vi "getLecServerCount.vi"(8 "error in (no error)":errorcluster, 11 "SM1000-control in":T1) -> (0 "error out":errorcluster, 2 "piServerCount":i32, 3 "SM1000-control out":T1)   [LabVIEW 2013, in "EC1000-control.lvlib" / "SM1000-control.lvclass"]
doc: "Get embedded controller device data.\n\nOnce a connection to the broadcast mechanism has been established, broadcast messages are then received and a table of available modules is built by the API. This method returns the number of distinct EC1000 modules that have transmitted valid broadcast packets since the 'clientAttachBroadcast' method was called.\nBecause of the asynchronous and periodic nature of the broadcast transmissions, it may take some time before all EC1000 controllers are recognized and reported via this method. Several successive calls may yield different results until enough time has passed to account for the longest broadcast interval. The broadcast interval is configured using the 'Session.requestFixedData' and 'Session.setFixedData' methods with the 'AdminConfig' data as an argument."
uses:
  SM1000-control.lvclass
  Object-reference.ctl
  SM1000-control.lvclass/SM1000-control.ctl
  Custom-errors.ctl
  C:/Users/vangeste/Desktop/Libraries/EC1000-control/LECBroadcast.dll
  LECBroadcast.dll
  DOTNET-error-int.vi
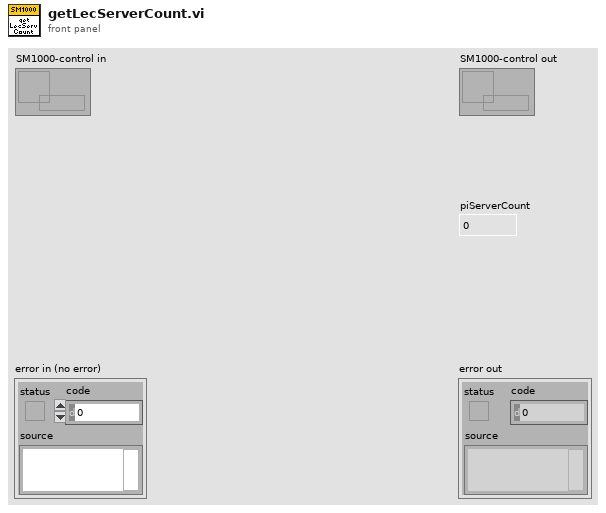
[diagram p1: front panel]
types:
  T1 = typedef "EC1000-control.lvlib/SM1000-control.lvclass/Object-reference.ctl" = refnum<data-value>
  T2 = typedef "EC1000-control.lvlib/SM1000-control.lvclass/Custom-errors.ctl" = enum16{"No error", "Not implemented", "Command not recognized", "Invalid input", "No connection", "Timeout", "Resource not loaded"}
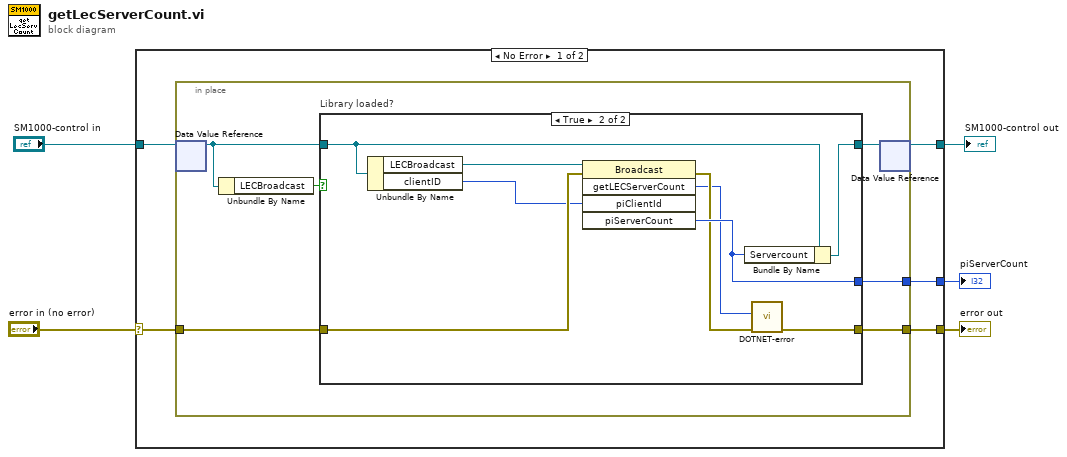
[diagram p0: block diagram]
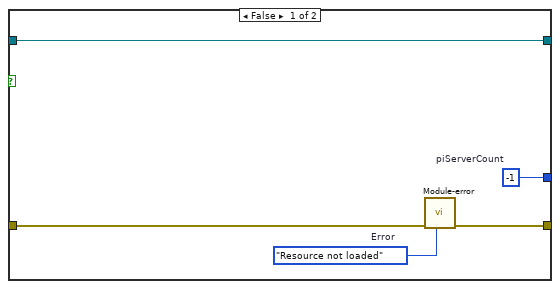
[diagram p2: hidden frame]
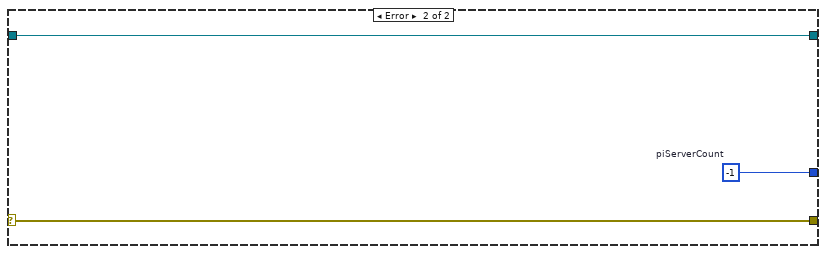
[diagram p3: hidden frame]
diagram:
  n1 = case shown="No Error" "error in (no error)" {
    selector: "error in (no error)" -> [w8 w33]
    tunnel: [w7 w33] -> w4
    tunnel: [w9 w32] -> w2
    tunnel: "SM1000-control in" -> [w10 w32]
    tunnel: [w6 w31] -> w1
    frame No Error {
      n2 = in-place {
        in-place-border: w8 -> [w16]
        in-place-border: [w13] -> w7
        in-place-border: [w11] -> w6
        n3 = in-place-dvr #1(w10) -> (w14:refnum<class "SM1000-control.lvclass">)  [unwired: 1 out]
        n4 = Unbundle By Name(w14) -> ("LECBroadcast"=w15:bool)
        n5 = case "Library loaded?" shown="True" w15 {
          tunnel: w16 -> [w21 w28]
          tunnel: w14 -> [w19 w30]
          tunnel: [w20 w24] -> w13
          tunnel: [w19 w27] -> w12
          tunnel: [w18 w25] -> w11
          frame False {
            w18 = -1  # piServerCount
            w17 = Custom-errors."Resource not loaded"  # Error
            n6 = call "Module-error.vi"("Error"=w17, "error in (no error)"=w21) -> ("error out"=w20:errorcluster)  [unwired: 9 in]
          }
          frame True {
            n7 = Unbundle By Name(w30) -> ("LECBroadcast"=w29:refnum<k24>, "clientID"=w26:i32)
            n8 = invoke class="Broadcast" method="getLECServerCount"(reference=w29, error in=w28, "piClientId"=w26) -> (error out=w23:errorcluster, "getLECServerCount"=w22:u32, "piServerCount"=w25:i32)  [unwired: 2 in, 2 out]
            n9 = Bundle By Name(cluster=w30, "Servercount"=w25) -> (w27:refnum<class "SM1000-control.lvclass">)
            n10 = call-poly "DOTNET-error.vi"("error in (no error)"=w23, "Retun code"=w22) -> ("error out"=w24:errorcluster)  [unwired: 9 in]
          }
        }
        n11 = in-place-dvr #1(w12) -> (w9:T1)  [unwired: 1 out]
      }
    }
    frame Error {
      w31 = -1  # piServerCount
    }
  }
  "error out" <- w4
  "SM1000-control out" <- w2
  "piServerCount" <- w1
